vi "6_6_19.vi"() -> ()   [LabVIEW 2018]
uses:
  <vilib>/Utility/file.llb/Read Delimited Spreadsheet (DBL).vi
  <vilib>/Analysis/NI_AALPro.lvlib
panel:
  out "heading":dbl
  out "df":dbl
  out "Length of Sample":dbl
  out "phase1 4":dbl format="%0.4f"
  out "phase1 3":dbl format="%0.4f"
  out "phase1 2":dbl format="%0.4f"
  out "phase1":dbl format="%0.4f"
  out "Waveform Graph 7":cluster{dbl, dbl, "all rows":dbl[]}(graph)
  out "Phase 4":cluster{dbl, dbl, "all rows":dbl[]}(graph)
  out "Amplitude spectrum 4":cluster{dbl, dbl, "all rows":dbl[]}(graph)
  out "est frequency peak 4":dbl format="%0.4f"
  out "Waveform Graph 8":cluster{dbl, dbl, "all rows":dbl[]}(graph)
  out "Phase 3":cluster{dbl, dbl, "all rows":dbl[]}(graph)
  out "Amplitude spectrum 3":cluster{dbl, dbl, "all rows":dbl[]}(graph)
  out "est frequency peak 3":dbl format="%0.4f"
  out "Waveform Graph 6":cluster{dbl, dbl, "all rows":dbl[]}(graph)
  out "Phase 2":cluster{dbl, dbl, "all rows":dbl[]}(graph)
  out "Amplitude spectrum 2":cluster{dbl, dbl, "all rows":dbl[]}(graph)
  out "est frequency peak 2":dbl format="%0.4f"
  out "Waveform Graph 4":cluster{dbl, dbl, "all rows":dbl[]}(graph)
  in  "SR":dbl
  out "Waveform Graph":cluster{dbl, dbl, "all rows":dbl[]}(graph)
  in  "stop":bool
  out "Waveform Graph 2":cluster{dbl, dbl, "all rows":dbl[]}(graph)
  out "est frequency peak":dbl format="%0.4f"
  out "Amplitude spectrum":cluster{dbl, dbl, "all rows":dbl[]}(graph)
  out "Phase":cluster{dbl, dbl, "all rows":dbl[]}(graph)
  in  "number of rows (all:-1)":i32=200000
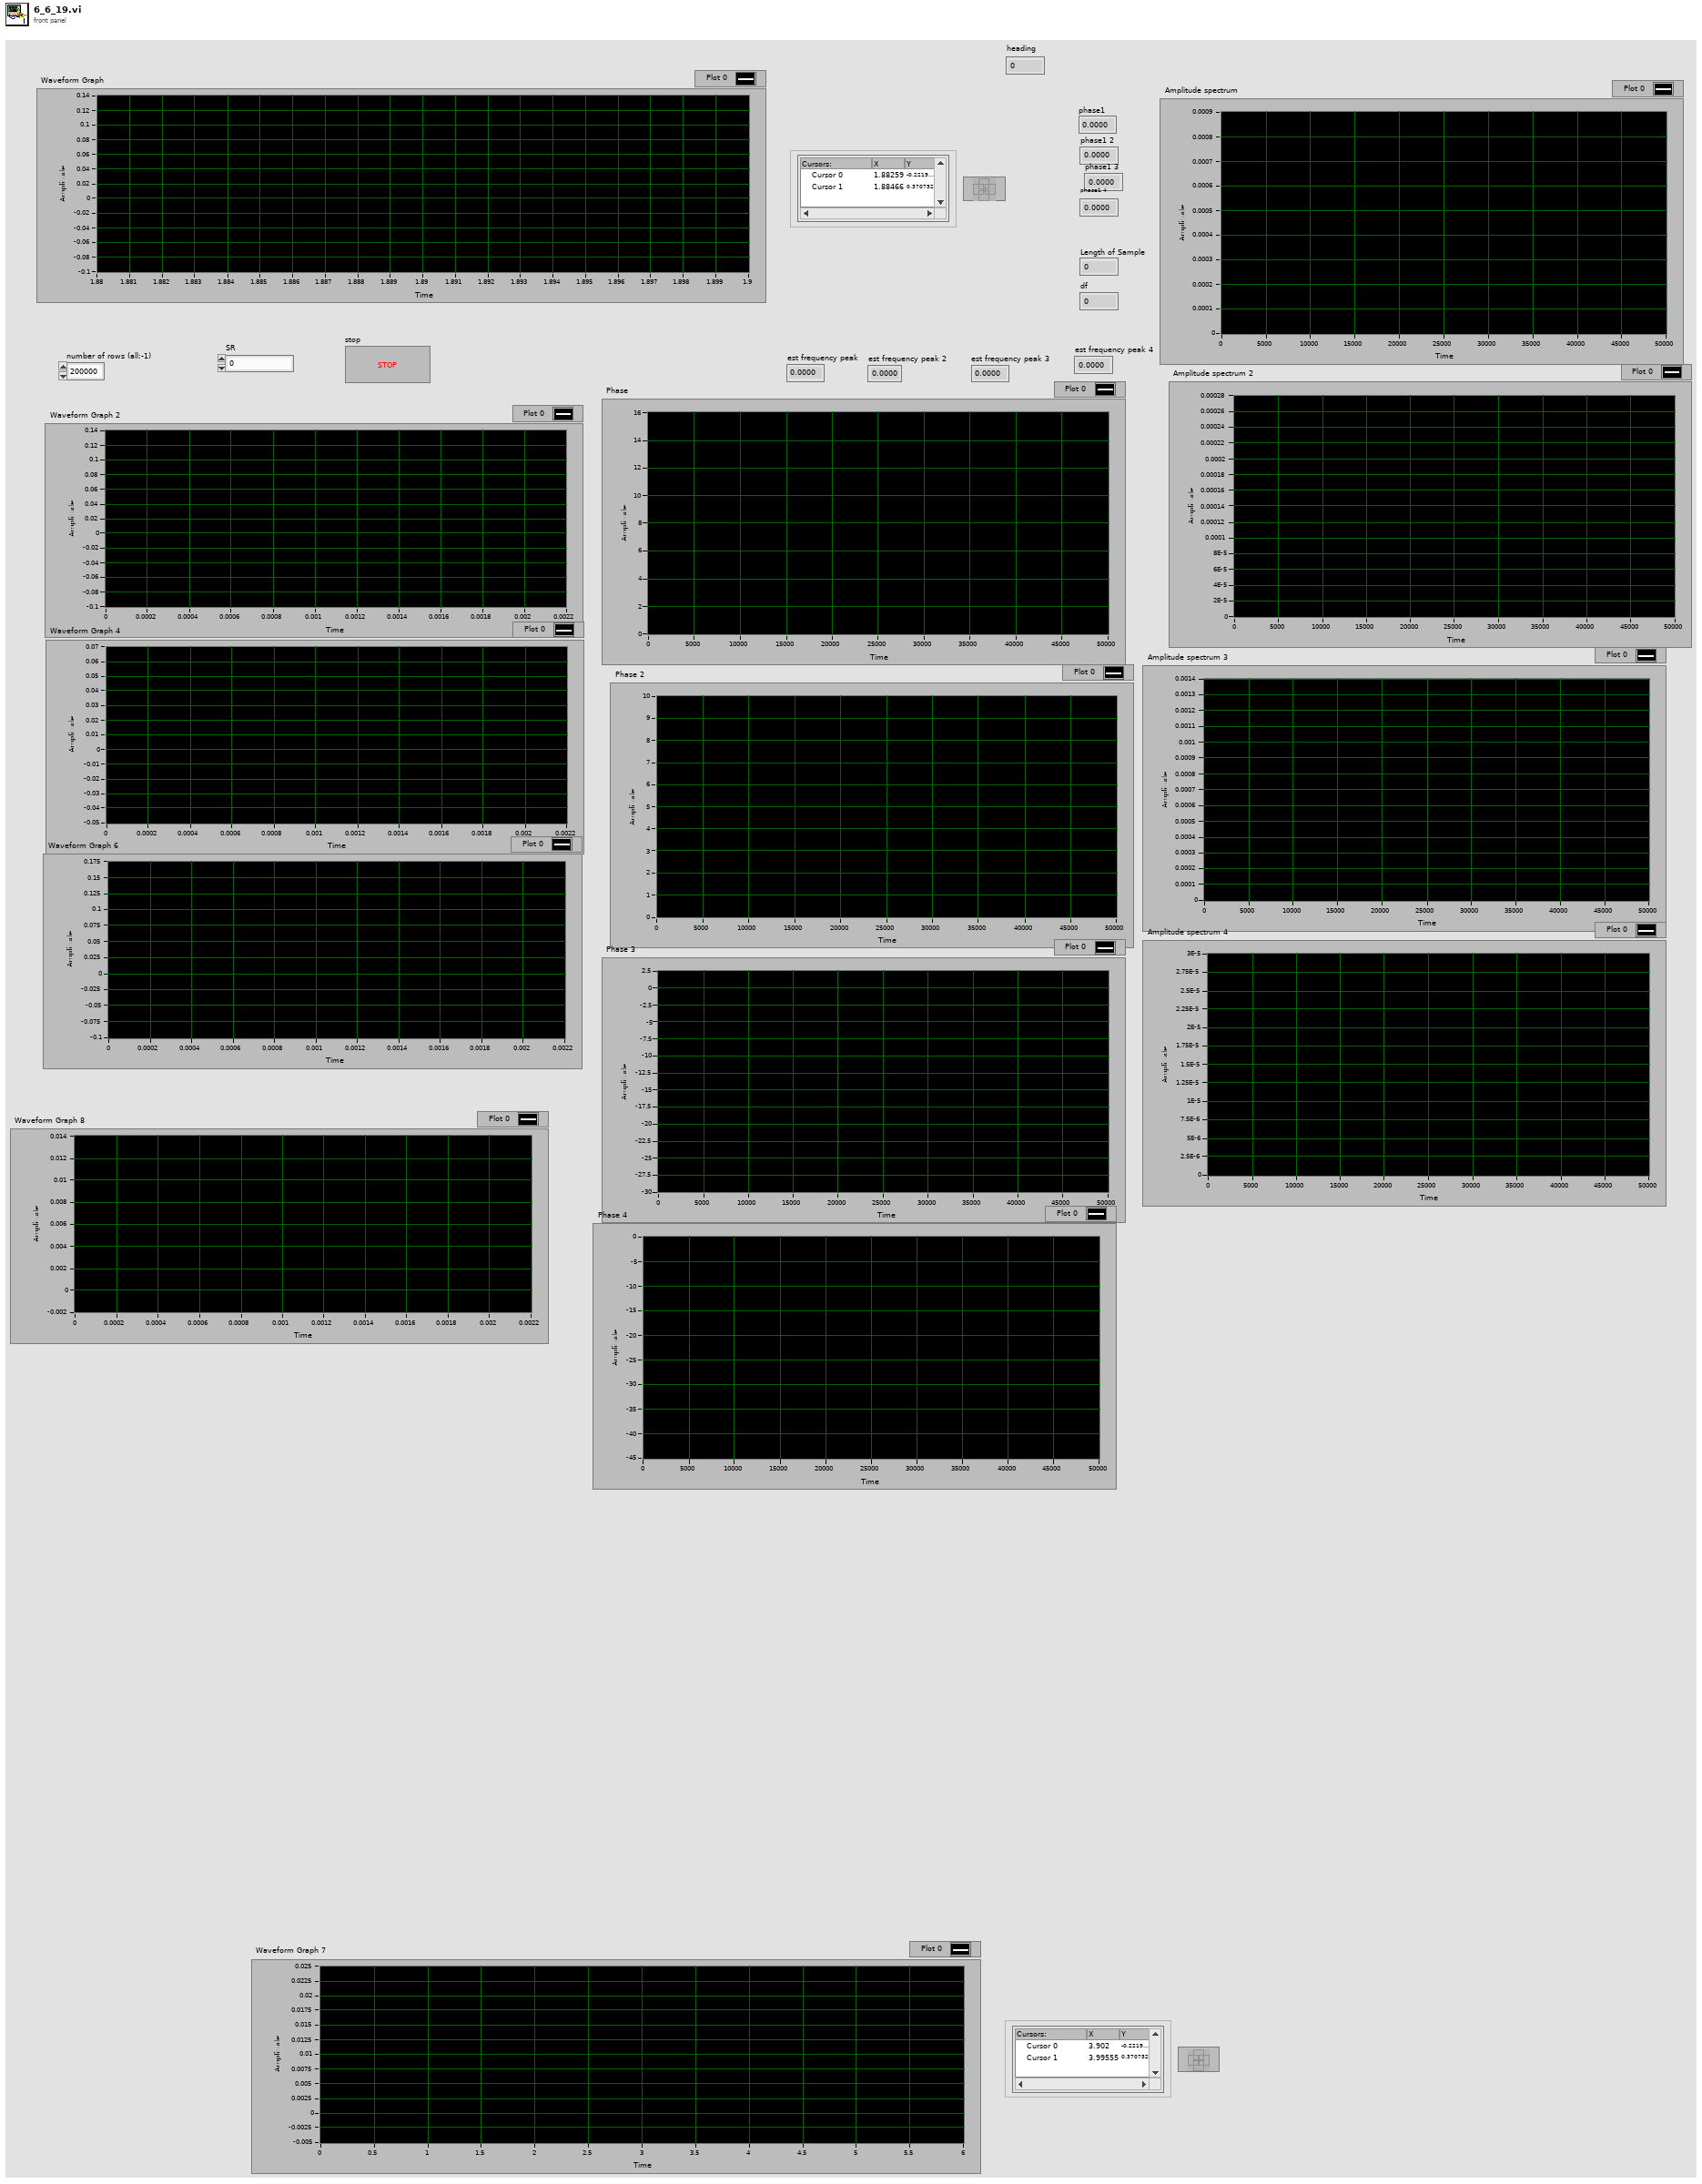
[diagram p1: front panel]
types:
  T1 = cluster{dbl, "df":dbl, "Power Spectrum (V^2 rms)":dbl[]}
  T2 = cluster{dbl, "df":dbl, "Amp Spectrum Phase (radians)":dbl[]}
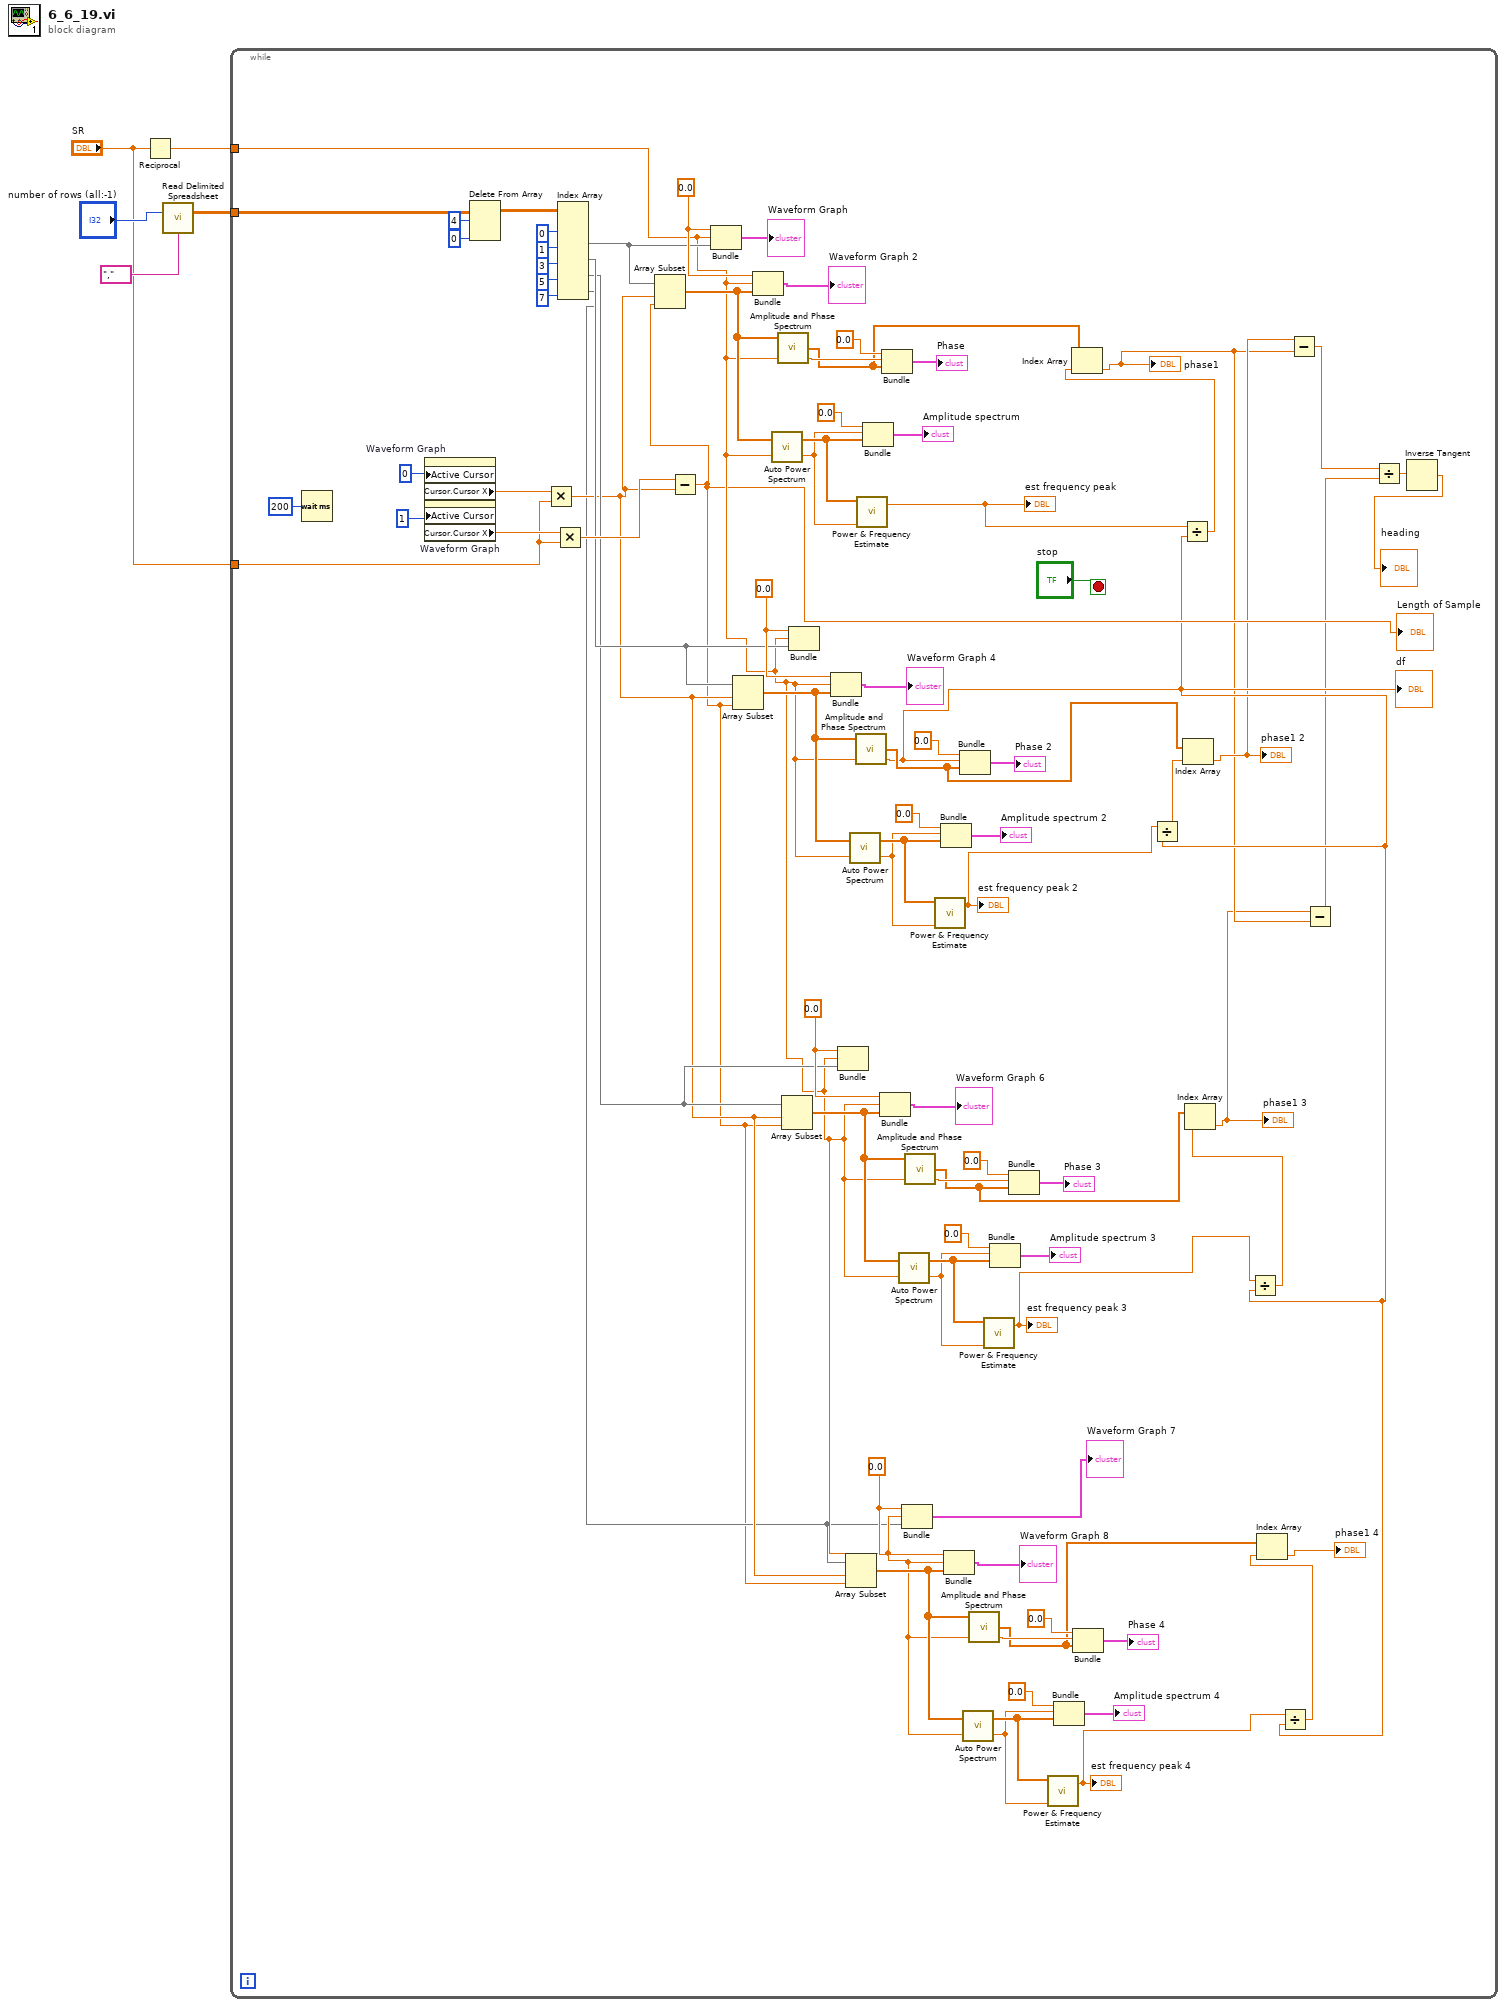
[diagram p0: block diagram]
diagram:
  n1 = Reciprocal(x="SR") -> (1/x=w2:dbl)
  n2 = call-poly <vilib>:"Read Delimited Spreadsheet.vi"("number of rows (all:-1)"="number of rows (all:-1)", "delimiter (\\t)"="," ("delimiter (\\t)")) -> ("all rows"=w4:dbl[][])  [unwired: 8 in, 5 out]
  n3 = while {
    tunnel: w4 -> [w91]
    tunnel: w2 -> [w30]
    tunnel: "SR" -> [w72]
    stop <- "stop" stop-if-true
    w41 = 0.0
    w52 = 0.0
    w62 = 0.0
    w77 = 0.0
    n4 = Wait (ms)(milliseconds to wait=u32 200) -> ()  [unwired: 1 out]
    n5 = property on="Waveform Graph" class="WFGraph (strict)"("Active Cursor"=u32 0) -> ("Cursor.Cursor X"=w74:dbl)  [unwired: 2 in, 2 out]
    n6 = property on="Waveform Graph" class="WFGraph (strict)"("Active Cursor"=u32 1) -> ("Cursor.Cursor X"=w73:dbl)  [unwired: 2 in, 2 out]
    n7 = Delete From Array(array=w91, length=4, index (row)=0) -> (array with subset deleted=w88:dbl[][])  [unwired: 1 in, 1 out]
    n8 = Multiply(x=w74, y=w72) -> (x*y=w31:dbl)
    n9 = Multiply(x=w73, y=w72) -> (x*y=w71:dbl)
    n10 = Index Array(array=w88, index (col) #1=0 ("index (row)"), index (col) #2=1 ("index (row)"), index (col) #3=3 ("index (row)"), index (col) #4=5 ("index (row)"), index (col) #5=7 ("index (row)")) -> (element #2=w75:dbl[], element #3=w53:dbl[], element #4=w42:dbl[], element #5=w29:dbl[])  [unwired: 5 in, 1 out]
    n11 = Subtract(x=w71, y=w31) -> (x-y=w22:dbl)
    "Length of Sample" <- w22
    n12 = Array Subset(array=w75, index=w31, length=w22) -> (w66:dbl[])
    n13 = Bundle(w77, w30, "all rows"=w75) -> (→"Waveform Graph":cluster{dbl, dbl, "all rows":dbl[]})  [unwired: 1 in]
    n14 = Array Subset(array=w53, index=w31, length=w22) -> (w56:dbl[])
    n15 = Bundle(w77, w30, w66) -> (→"Waveform Graph 2":cluster{dbl, dbl, dbl[]})  [unwired: 1 in]
    n16 = call <vilib>:"Auto Power Spectrum.vi"("dt"=w30, "Signal (V)"=w66) -> ("df"=w69:dbl, "Power Spectrum (V^2 rms)"=w70:dbl[])
    n17 = call <vilib>:"Amplitude and Phase Spectrum.vi"("dt"=w30, "Signal (V)"=w66) -> ("df"=w64:dbl, "Amp Spectrum Phase (radians)"=w27:dbl[])  [unwired: 1 in, 1 out]
    n18 = Array Subset(array=w42, index=w31, length=w22) -> (w46:dbl[])
    n19 = Bundle(w62, w30, "all rows"=w53) -> ()  [unwired: 1 in, 1 out]
    n20 = Bundle(w62, w30, w56) -> (→"Waveform Graph 4":cluster{dbl, dbl, dbl[]})  [unwired: 1 in]
    n21 = Bundle(w52, w30, "all rows"=w42) -> ()  [unwired: 1 in, 1 out]
    n22 = Array Subset(array=w29, index=w31, length=w22) -> (w35:dbl[])
    n23 = call <vilib>:"Auto Power Spectrum.vi"("dt"=w30, "Signal (V)"=w56) -> ("df"=w59:dbl, "Power Spectrum (V^2 rms)"=w60:dbl[])
    n24 = call <vilib>:"Amplitude and Phase Spectrum.vi"("dt"=w30, "Signal (V)"=w56) -> ("df"=w14:dbl, "Amp Spectrum Phase (radians)"=w26:dbl[])  [unwired: 1 in, 1 out]
    "df" <- w14
    n25 = call <vilib>:"Power & Frequency Estimate.vi"("df"=w69, "Power Spectrum (V^2 rms)"=w70) -> ("est frequency peak"=w15:dbl)  [unwired: 4 in, 1 out]
    "est frequency peak" <- w15
    n26 = Bundle(0.0, "df"=w69, "Power Spectrum (V^2 rms)"=w70) -> (→"Amplitude spectrum":T1)  [unwired: 1 in]
    n27 = Bundle(w52, w30, w46) -> (→"Waveform Graph 6":cluster{dbl, dbl, dbl[]})  [unwired: 1 in]
    n28 = Bundle(0.0, "df"=w64, "Amp Spectrum Phase (radians)"=w27) -> (→"Phase":T2)  [unwired: 1 in]
    n29 = call <vilib>:"Auto Power Spectrum.vi"("dt"=w30, "Signal (V)"=w46) -> ("df"=w49:dbl, "Power Spectrum (V^2 rms)"=w50:dbl[])
    n30 = Bundle(w41, w30, "all rows"=w29) -> (→"Waveform Graph 7":cluster{dbl, dbl, "all rows":dbl[]})  [unwired: 1 in]
    n31 = call <vilib>:"Amplitude and Phase Spectrum.vi"("dt"=w30, "Signal (V)"=w46) -> ("df"=w44:dbl, "Amp Spectrum Phase (radians)"=w25:dbl[])  [unwired: 1 in, 1 out]
    n32 = call <vilib>:"Power & Frequency Estimate.vi"("df"=w59, "Power Spectrum (V^2 rms)"=w60) -> ("est frequency peak"=w21:dbl)  [unwired: 4 in, 1 out]
    "est frequency peak 2" <- w21
    n33 = Bundle(0.0, "df"=w59, "Power Spectrum (V^2 rms)"=w60) -> (→"Amplitude spectrum 2":T1)  [unwired: 1 in]
    n34 = Bundle(w41, w30, w35) -> (→"Waveform Graph 8":cluster{dbl, dbl, dbl[]})  [unwired: 1 in]
    n35 = Bundle(0.0, "df"=w14, "Amp Spectrum Phase (radians)"=w26) -> (→"Phase 2":T2)  [unwired: 1 in]
    n36 = call <vilib>:"Auto Power Spectrum.vi"("dt"=w30, "Signal (V)"=w35) -> ("df"=w38:dbl, "Power Spectrum (V^2 rms)"=w39:dbl[])
    n37 = call <vilib>:"Amplitude and Phase Spectrum.vi"("dt"=w30, "Signal (V)"=w35) -> ("df"=w33:dbl, "Amp Spectrum Phase (radians)"=w23:dbl[])  [unwired: 1 in, 1 out]
    n38 = call <vilib>:"Power & Frequency Estimate.vi"("df"=w49, "Power Spectrum (V^2 rms)"=w50) -> ("est frequency peak"=w19:dbl)  [unwired: 4 in, 1 out]
    "est frequency peak 3" <- w19
    n39 = Bundle(0.0, "df"=w49, "Power Spectrum (V^2 rms)"=w50) -> (→"Amplitude spectrum 3":T1)  [unwired: 1 in]
    n40 = Bundle(0.0, "df"=w44, "Amp Spectrum Phase (radians)"=w25) -> (→"Phase 3":T2)  [unwired: 1 in]
    n41 = call <vilib>:"Power & Frequency Estimate.vi"("df"=w38, "Power Spectrum (V^2 rms)"=w39) -> ("est frequency peak"=w17:dbl)  [unwired: 4 in, 1 out]
    "est frequency peak 4" <- w17
    n42 = Bundle(0.0, "df"=w38, "Power Spectrum (V^2 rms)"=w39) -> (→"Amplitude spectrum 4":T1)  [unwired: 1 in]
    n43 = Bundle(0.0, "df"=w33, "Amp Spectrum Phase (radians)"=w23) -> (→"Phase 4":T2)  [unwired: 1 in]
    n44 = Divide(x=w21, y=w14) -> (x/y=w20:dbl)
    n45 = Divide(x=w15, y=w14) -> (x/y=w13:dbl)
    n46 = Index Array(array=w27, index=w13) -> (element=w11:dbl)
    "phase1" <- w11
    n47 = Index Array(array=w26, index=w20) -> (element=w12:dbl)
    "phase1 2" <- w12
    n48 = Divide(x=w19, y=w14) -> (x/y=w18:dbl)
    n49 = Index Array(array=w25, index=w18) -> (element=w10:dbl)
    "phase1 3" <- w10
    n50 = Divide(x=w17, y=w14) -> (x/y=w16:dbl)
    n51 = Index Array(array=w23, index=w16) -> (element=→"phase1 4":dbl)
    n52 = Subtract(x=w12, y=w11) -> (x-y=w9:dbl)
    n53 = Subtract(x=w10, y=w11) -> (x-y=w8:dbl)
    n54 = Divide(x=w9, y=w8) -> (x/y=w7:dbl)
    n55 = Inverse Tangent(1:w7) -> (0:→"heading":dbl)
  }
